vi "Generate_WayPoints_Hopping WITH VariablePauseTim2.vi"(11 "Input Cluster":T2={"Scan Rate (um/s)"=15.0, "X Start"=15.0, "X End"=15.0, "Y Start"=15.0, "Y End"=15.0, " Z Start"=15.0, "HoppingDistance"=1.0, "Voltage1"=15.0, "Z End"=15.0, "Approach Rate Hopping (um/s)"=15.0, "Retrack Rate (um/s)"=15.0, "Voltage2"=15.0, "Approach Rate (um/s)"=15.0, "Hold Time START / s"=15.0, "Hold Time Delta / s"=15.0, "Voltage1 During Retract"=0.0, "Pause on First Approach?"=FALSE, "Voltage2 During Retract"=0.0, "Voltage1 During Hold Time"=0.0, "Voltage2 During Hold Time"=0.0, "Update position loop wait time (us)"=0}) -> (1 "output cluster":T1)   [LabVIEW 2023]
uses:
  TypeDefs/WayPointCluster.ctl
  User_Vi/Settings.vi
panel:
  in  "WayPointCluster":T1
  out "Y  P":dbl
  out "X  P":dbl
  out "HoppingDistanceX":dbl
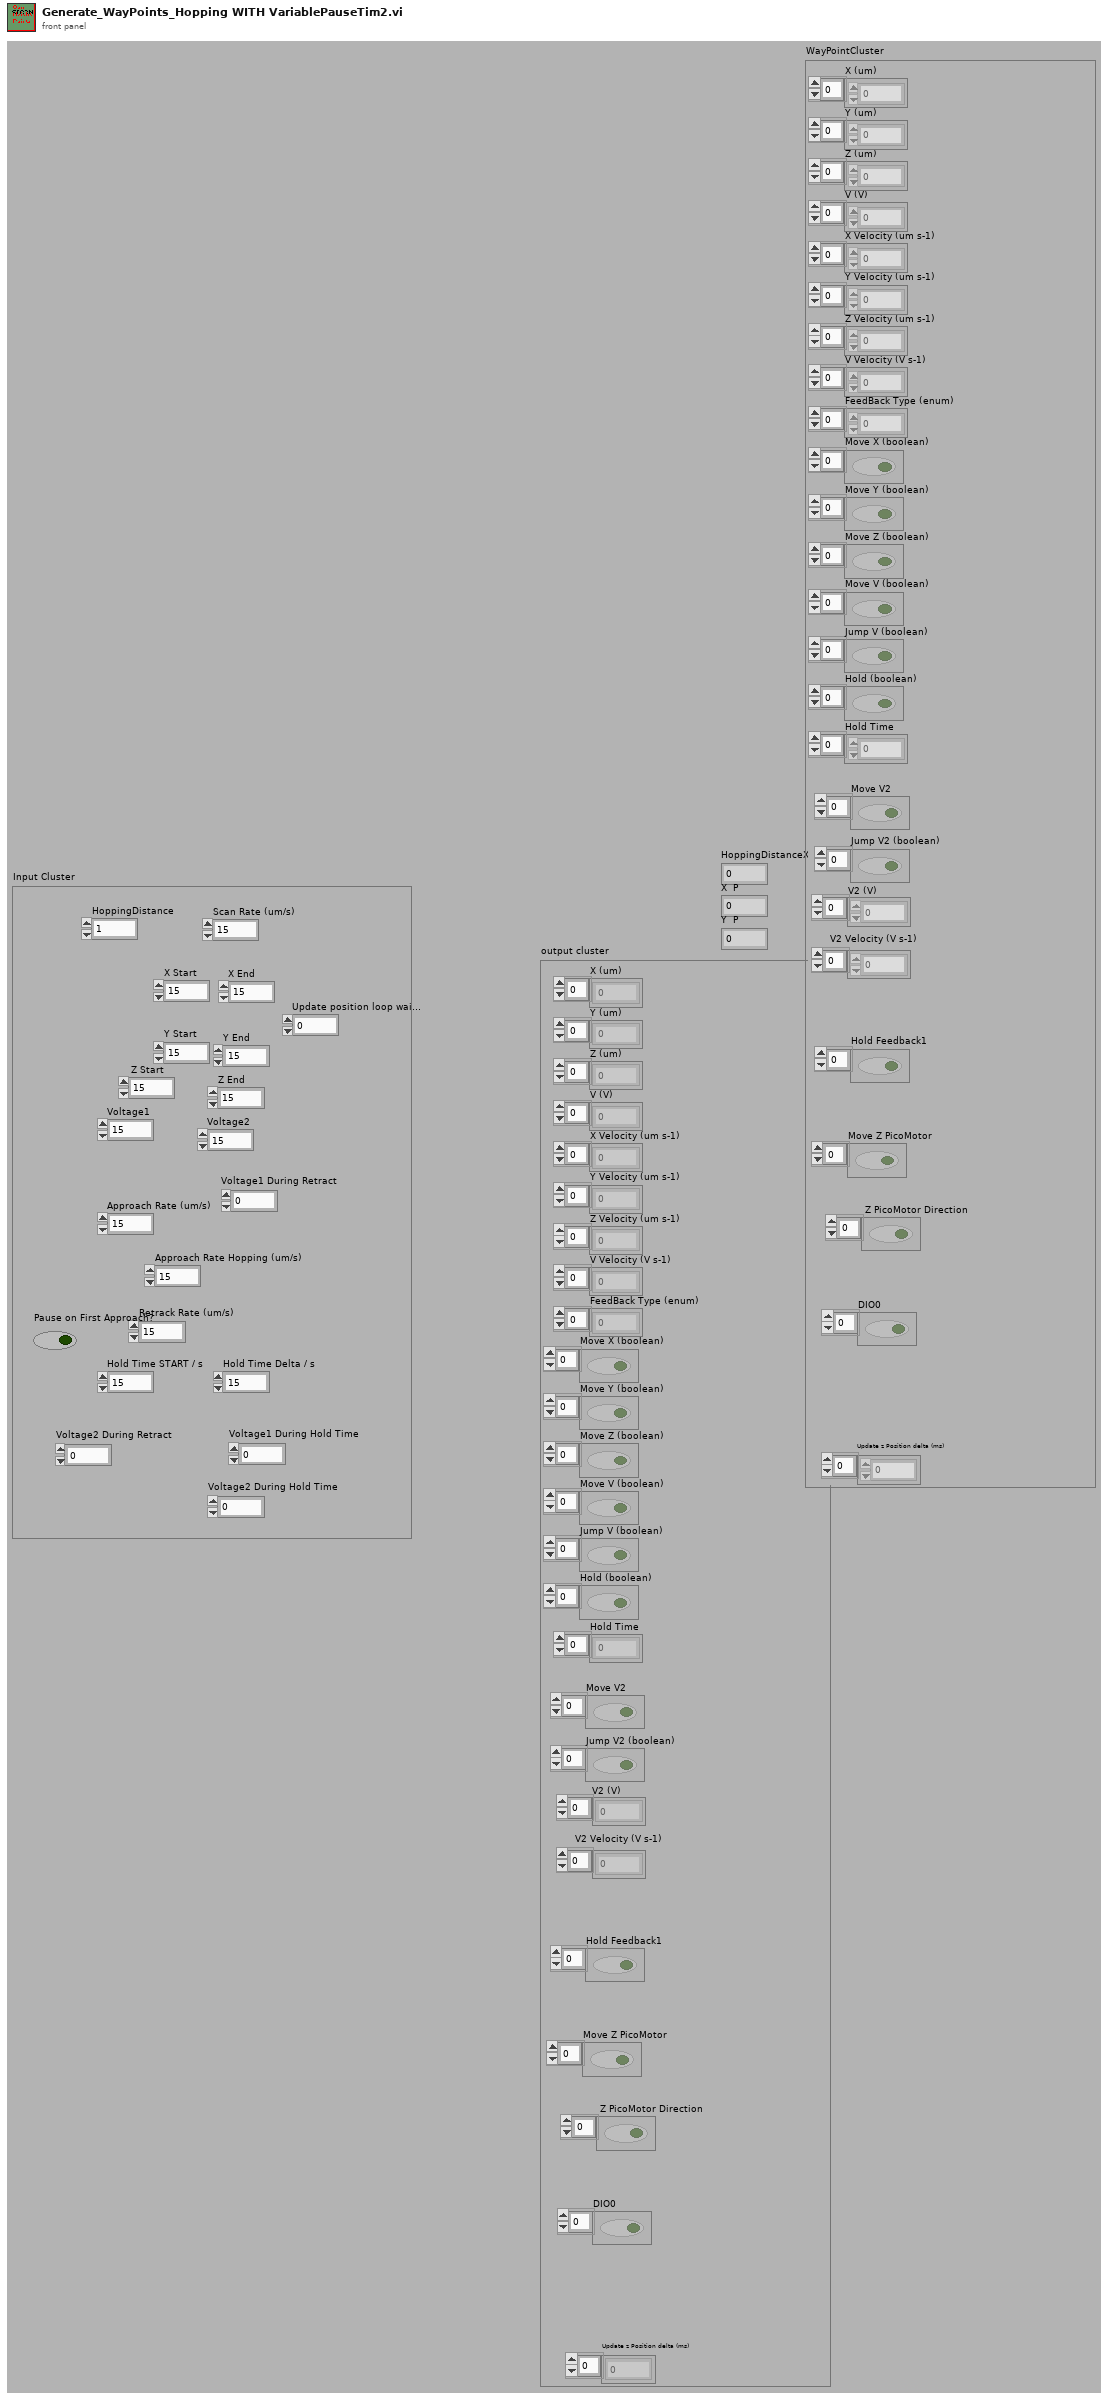
[diagram p1: front panel]
types:
  T1 = typedef "WayPointCluster.ctl" = cluster{"X (um)":dbl[], "Y (um)":dbl[], "Z (um)":dbl[], "V (V)":dbl[], "X Velocity (um s-1)":dbl[], "Y Velocity (um s-1)":dbl[], "Z Velocity (um s-1)":dbl[], "V Velocity (V s-1)":dbl[], "FeedBack Type (enum)":u16[], "Move X (boolean)":bool[], "Move Y (boolean)":bool[], "Move Z (boolean)":bool[], "Move V (boolean)":bool[], "Jump V (boolean)":bool[], "Hold (boolean)":bool[], "Hold Time":u32[], "V2 (V)":dbl[], "Move V2":bool[], "V2 Velocity (V s-1)":dbl[], "Jump V2 (boolean)":bool[], "Update z Position delta (ms)":i16[], "Hold Feedback1":bool[], "Move Z PicoMotor":bool[], " Z PicoMotor Direction":bool[], "DIO0":bool[]}
  T2 = cluster{"Scan Rate (um/s)":dbl, "X Start":dbl, "X End":dbl, "Y Start":dbl, "Y End":dbl, " Z Start":dbl, "HoppingDistance":dbl, "Voltage1":dbl, "Z End":dbl, "Approach Rate Hopping (um/s)":dbl, "Retrack Rate (um/s)":dbl, "Voltage2":dbl, "Approach Rate (um/s)":dbl, "Hold Time START / s":dbl, "Hold Time Delta / s":dbl, "Voltage1 During Retract":dbl, "Pause on First Approach?":bool, "Voltage2 During Retract":dbl, "Voltage1 During Hold Time":dbl, "Voltage2 During Hold Time":dbl, "Update position loop wait time (us)":u32}
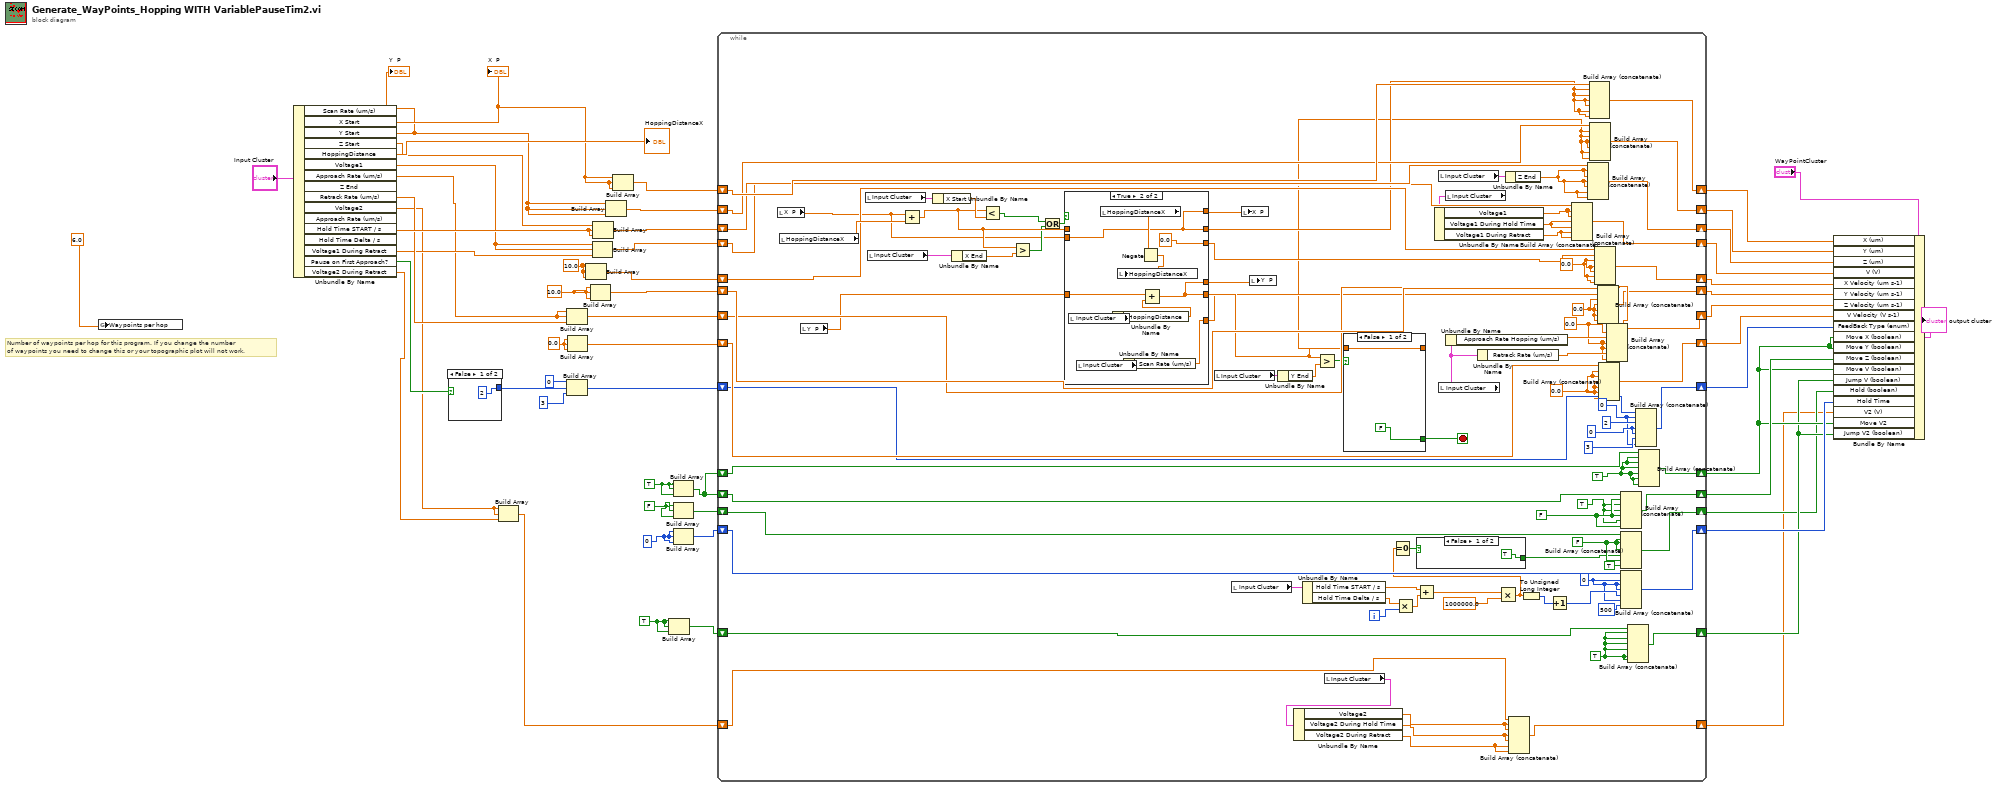
[diagram p0: block diagram]
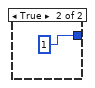
[diagram p2: hidden frame]
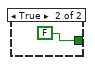
[diagram p3: hidden frame]
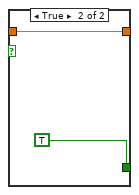
[diagram p4: hidden frame]
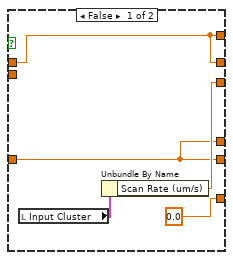
[diagram p5: hidden frame]
diagram:
  w18 = TRUE
  w19 = u32 0 ("element")
  w20 = FALSE
  w21 = TRUE
  w14 = 10.0 ("element")
  w15 = 10.0 ("element")
  w17 = 0.0 ("element")
  # "Number of waypoints per hop for this program. If you change the number\nof waypoints you need to change this or your topographic plot will not work."
  n1 = global write "Settings.vi" "Waypoints per hop"(6.0) -> ()
  n2 = Unbundle By Name("Input Cluster") -> ("X Start"=w35:dbl, "Y Start"=w34:dbl, "Z Start"=w36:dbl, "HoppingDistance"=→"HoppingDistanceX":dbl, "Voltage1"=w32:dbl, "Approach Rate (um/s)"=w16:dbl, "Z End"=w33:dbl, "Retrack Rate (um/s)"=w31:dbl, "Voltage2"=w8:dbl, "Voltage1 During Retract"=w23:dbl, "Pause on First Approach?"=w11:bool, "Voltage2 During Retract"=w7:dbl)  [unwired: 4 out]
  "X  P" <- w35
  "Y  P" <- w34
  n3 = case shown="False" w11 {
    tunnel: [u16 2 ("element") u16 1 ("element")] -> w10
    frame False {
    }
    frame True {
    }
  }
  n4 = Build Array(w8, w8, w7) -> (w4:dbl[])
  n5 = Build Array(w16, w16, w31) -> (w43:dbl[])
  n6 = Build Array(u16 0 ("element"), w10, u16 3 ("element")) -> (w39:u16[])
  n7 = Build Array(w17, w17, w17) -> (w41:dbl[])
  n8 = Build Array(w14, w14, w14) -> (w46:dbl[])
  n9 = Build Array(w15, w15, w15) -> (w45:dbl[])
  n10 = Build Array(w32, w32, w23) -> (w48:dbl[])
  n11 = Build Array(w36, w33, w33) -> (w50:dbl[])
  n12 = Build Array(w34, w34, w34) -> (w52:dbl[])
  n13 = Build Array(w35, w35, w35) -> (w54:dbl[])
  n14 = Build Array(w18, w18, w18) -> (w25:bool[])
  n15 = Build Array(w21, w21, w21) -> (w24:bool[])
  n16 = Build Array(w20, w20, w20) -> (w28:bool[])
  n17 = Build Array(w19, w19, w19) -> (w27:u32[])
  n18 = while {
    shift-right: [w146] -> w53
    shift-left: w54 -> [w147]
    shift-right: [w138] -> w51
    shift-left: w52 -> [w128]
    shift-right: [w137] -> w49
    shift-left: w50 -> [w145]
    shift-right: [w136] -> w47
    shift-left: w48 -> [w144]
    shift-right: [w135] -> w29
    shift-left: w46 -> [w143]
    shift-right: [w134] -> w44
    shift-left: w45 -> [w142]
    shift-right: [w133] -> w42
    shift-left: w43 -> [w141]
    shift-right: [w132] -> w40
    shift-left: w41 -> [w140]
    shift-right: [w131] -> w38
    shift-left: w39 -> [w139]
    shift-right: [w102] -> w9
    shift-left: w24 -> [w101]
    shift-right: [w103] -> w2
    shift-left: w28 -> [w107]
    shift-right: [w104] -> w26
    shift-left: w27 -> [w106]
    shift-right: [w99] -> w5
    shift-left: w25 -> [w100]
    shift-right: [w93] -> w6
    shift-left: w24 -> [w94]
    shift-right: [w76] -> w1
    shift-left: w4 -> [w77]
    i -> [w96]
    stop <- w118 stop-if-true
    w65 = TRUE
    w61 = TRUE
    w86 = u32 0 ("element")
    w88 = FALSE
    w64 = FALSE
    w58 = TRUE
    w66 = u16 0 ("element")
    w69 = 0.0 ("element")
    w70 = 0.0 ("element")
    w67 = 0.0 ("element")
    w68 = 0.0 ("element")
    w59 = u16 0 ("element")
    n19 = local read "X  P"() -> (w116:dbl)
    n20 = local read "HoppingDistanceX"() -> (w148:dbl)
    n21 = local read "Y  P"() -> (w115:dbl)
    n22 = local read "Input Cluster"() -> (w150:T2)
    n23 = local read "Input Cluster"() -> (w149:T2)
    n24 = Add(x=w116, y=w148) -> (x+y=w124:dbl)
    n25 = Unbundle By Name(w150) -> ("X Start"=w127:dbl)
    n26 = Unbundle By Name(w149) -> ("X End"=w125:dbl)
    n27 = Less?(x=w124, y=w127) -> (x < y?=w126:bool)
    n28 = Greater?(x=w124, y=w125) -> (0:w123:bool)
    n29 = Or(x=w126, y=w123) -> (x .or. y?=w122:bool)
    n30 = case shown="True" w122 {
      tunnel: w124 -> [w157 _]
      tunnel: [w157 w163] -> w74
      tunnel: w116 -> [_ w163]
      tunnel: w115 -> [w158 w164]
      tunnel: [w158 w162] -> w114
      tunnel: [w160 0.0] -> w109
      tunnel: [0.0 w165] -> w108
      tunnel: [w158 w162] -> w113
      tunnel: [w157 w163] -> w112
      frame False {
        n31 = local read "Input Cluster"() -> (w161:T2)
        n32 = Unbundle By Name(w161) -> ("Scan Rate (um/s)"=w160:dbl)
      }
      frame True {
        n33 = local read "Input Cluster"() -> (w169:T2)
        n34 = local read "Input Cluster"() -> (w167:T2)
        n35 = local read "HoppingDistanceX"() -> (w171:dbl)
        n36 = Unbundle By Name(w169) -> ("HoppingDistance"=w168:dbl)
        n37 = Unbundle By Name(w167) -> ("Scan Rate (um/s)"=w165:dbl)
        n38 = Negate(x=w171) -> (-x=w170:dbl)
        n39 = local write "HoppingDistanceX"(w170) -> ()
        n40 = Add(x=w164, y=w168) -> (x+y=w162:dbl)
      }
    }
    n41 = local read "Input Cluster"() -> (w121:T2)
    n42 = local read "Input Cluster"() -> (w105:T2)
    n43 = local write "X  P"(w112) -> ()
    n44 = local write "Y  P"(w113) -> ()
    n45 = Unbundle By Name(w121) -> ("Y End"=w120:dbl)
    n46 = Unbundle By Name(w105) -> ("Hold Time START / s"=w83:dbl, "Hold Time Delta / s"=w98:dbl)
    n47 = Greater?(x=w114, y=w120) -> (0:w119:bool)
    n48 = local read "Input Cluster"() -> (w79:T2)
    n49 = Unbundle By Name(w79) -> ("Voltage2"=w75:dbl, "Voltage2 During Hold Time"=w78:dbl, "Voltage2 During Retract"=w60:dbl)
    n50 = case shown="False" w119 {
      tunnel: w114 -> [w154 w156]
      tunnel: [w154 w156] -> w73
      tunnel: [FALSE TRUE] -> w118
      frame False {
      }
      frame True {
      }
    }
    n51 = Multiply(x=w98, y=w96) -> (x*y=w97:dbl)
    n52 = Add(x=w83, y=w97) -> (x+y=w95:dbl)
    n53 = local read "Input Cluster"() -> (w130:T2)
    n54 = local read "Input Cluster"() -> (w117:T2)
    n55 = local read "Input Cluster"() -> (w129:T2)
    n56 = Unbundle By Name(w129) -> ("Voltage1"=w81:dbl, "Voltage1 During Hold Time"=w80:dbl, "Voltage1 During Retract"=w71:dbl)
    n57 = Unbundle By Name(w117) -> ("Approach Rate Hopping (um/s)"=w110:dbl)
    n58 = Unbundle By Name(w117) -> ("Retrack Rate (um/s)"=w90:dbl)
    n59 = Multiply(x=w95, y=1000000.0) -> (x*y=w82:dbl)
    n60 = Equal To 0?(x=w82) -> (x = 0?=w84:bool)
    n61 = case shown="False" w84 {
      tunnel: [TRUE FALSE] -> w85
      frame False {
      }
      frame True {
      }
    }
    n62 = Unbundle By Name(w130) -> ("Z End"=w72:dbl)
    n63 = Build Array (concatenate)(w77, w75, w75, w78, w78, w60, w60) -> (w76:dbl[])
    n64 = To Unsigned Long Integer(number=w82) -> (unsigned 32bit integer=w91:u32)
    n65 = Increment(x=w91) -> (x+1=w87:u32)
    n66 = Build Array (concatenate)(w144, w81, w81, w80, w80, w71, w71) -> (w136:dbl[])
    n67 = Build Array (concatenate)(w145, w72, w72, w72, w72, w72, w72) -> (w137:dbl[])
    n68 = Build Array (concatenate)(w147, w74, w74, w74, w74, w74, w74) -> (w146:dbl[])
    n69 = Build Array (concatenate)(w128, w73, w73, w73, w73, w73, w73) -> (w138:dbl[])
    n70 = Build Array (concatenate)(w143, w109, w70, w70, w70, w70, w70) -> (w135:dbl[])
    n71 = Build Array (concatenate)(w142, w108, w69, w69, w69, w69, w69) -> (w134:dbl[])
    n72 = Build Array (concatenate)(w140, w67, w67, w67, w67, w67, w67) -> (w132:dbl[])
    n73 = Build Array (concatenate)(w141, w68, w110, w68, w68, w90, w68) -> (w133:dbl[])
    n74 = Build Array (concatenate)(w101, w64, w58, w58, w64, w58, w64) -> (w102:bool[])
    n75 = Build Array (concatenate)(w107, w88, w88, w88, w85, w88, TRUE ("element")) -> (w103:bool[])
    n76 = Build Array (concatenate)(w106, w86, w86, w86, w87, w86, u32 500 ("element")) -> (w104:u32[])
    n77 = Build Array (concatenate)(w100, w61, w61, w61, w61, w61, w61) -> (w99:bool[])
    n78 = Build Array (concatenate)(w139, w59, u16 2 ("element"), w66, w66, u16 3 ("element"), w59) -> (w131:u16[])
    n79 = Build Array (concatenate)(w94, w65, w65, w65, w65, w65, w65) -> (w93:bool[])
  }
  n80 = Bundle By Name(cluster="WayPointCluster", "X (um)"=w53, "Y (um)"=w51, "Z (um)"=w49, "V (V)"=w47, "X Velocity (um s-1)"=w29, "Y Velocity (um s-1)"=w44, "Z Velocity (um s-1)"=w42, "V Velocity (V s-1)"=w40, "FeedBack Type (enum)"=w38, "Move X (boolean)"=w6, "Move Y (boolean)"=w6, "Move Z (boolean)"=w9, "Move V (boolean)"=w6, "Jump V (boolean)"=w5, "Hold (boolean)"=w2, "Hold Time"=w26, "V2 (V)"=w1, "Move V2"=w6, "Jump V2 (boolean)"=w5) -> (→"output cluster":T1)
